vi "MLST.vi"(8 "error in (no error)":errorcluster, 10 "RemoteDirectory":string, 11 "FTP in":refnum<class "FTP.lvclass">) -> (0 "error out":errorcluster, 3 "FTP out":refnum<class "FTP.lvclass">)   [LabVIEW 2017, in "FTP_UpgradeCSMF.lvlib" / "FTP.lvclass"]
uses:
  FTP.lvclass
panel:
  out "Array":string[](array[string])
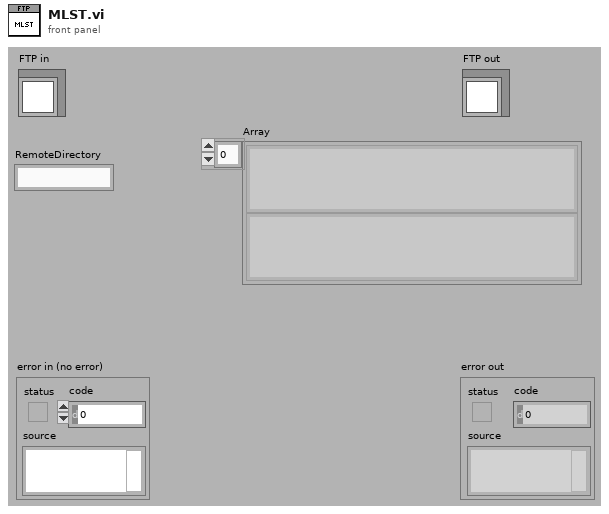
[diagram p1: front panel]
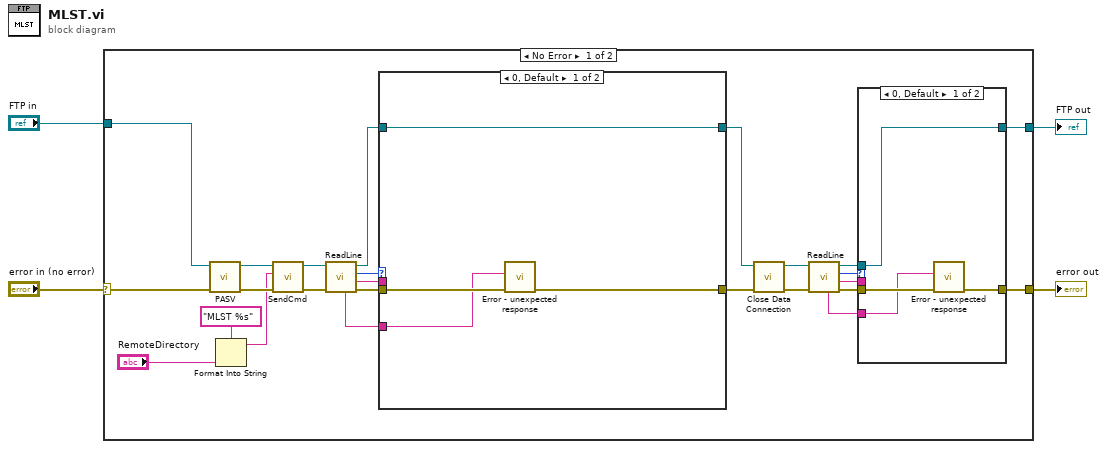
[diagram p0: block diagram]
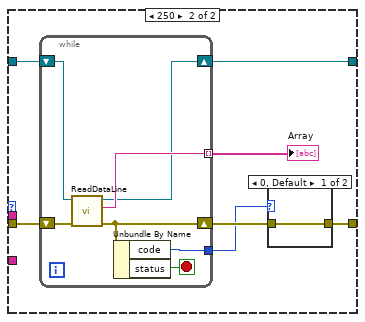
[diagram p3: hidden frame]
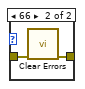
[diagram p4: hidden frame]
diagram:
  n1 = case shown="No Error" "error in (no error)" {
    selector: "error in (no error)" -> [w27 w58]
    tunnel: [w14 w58] -> w3
    tunnel: [w11 w57] -> w1
    tunnel: "FTP in" -> [w26 w57]
    frame No Error {
      n2 = call "PASV.vi"("error in (no error)"=w27, "FTP in"=w26) -> ("error out"=w24:errorcluster, "FTP out"=w25:refnum<class "FTP.lvclass">)  [unwired: 8 in]
      n3 = Format Into String(format string="MLST %s" ("cmd"), "RemoteDirectory") -> (resulting string=w8:string)  [unwired: 2 in, 1 out]
      n4 = call "SendCmd.vi"("error in (no error)"=w24, "cmd"=w8, "FTP in"=w25) -> ("error out"=w28:errorcluster, "FTP out"=w29:refnum<class "FTP.lvclass">)  [unwired: 7 in]
      n5 = call "ReadLine.vi"("error in (no error)"=w28, "FTP in"=w29) -> ("error out"=w23:errorcluster, "Line"=w21:string, "code"=w22:i32, "FTP out"=w20:refnum<class "FTP.lvclass">, "Full Line"=w5:string)  [unwired: 5 in]
      n6 = case shown="0, Default" w22 {
        tunnel: w23 -> [w38 w46]
        tunnel: w20 -> [w39 w45]
        tunnel: [w37 w43] -> w19
        tunnel: [w39 w42] -> w18
        tunnel: w21 -> [_ _]
        tunnel: w5 -> [w36 _]
        frame 0, Default {
          n7 = call "Error - unexpected response.vi"("error in (no error)"=w38, "Full Response"=w36) -> ("error out"=w37:errorcluster)  [unwired: 9 in]
        }
        frame 250 {
          n8 = while {
            tunnel: [w54] -> w44 mode=indexing
            shift-right: [w50] -> w41
            shift-left: w46 -> [w56]
            shift-right: [w51] -> w42
            shift-left: w45 -> [w55]
            tunnel: [w52] -> w40
            stop <- w53 stop-if-true
            n9 = call "ReadDataLine.vi"("error in (no error)"=w56, "FTP in"=w55) -> ("error out"=w50:errorcluster, "Data"=w54:string, "FTP out"=w51:refnum<class "FTP.lvclass">)  [unwired: 7 in]
            n10 = Unbundle By Name(w50) -> ("code"=w52:i32, "status"=w53:bool)
          }
          "Array" <- w44
          n11 = case shown="0, Default" w40 {
            tunnel: [w47 w49] -> w43
            tunnel: w41 -> [w47 w48]
            frame 0, Default {
            }
            frame 66 {
              n12 = call <vilib>:"Clear Errors.vi"("error in (no error)"=w48) -> ("error out"=w49:errorcluster)  [unwired: 5 in, 1 out]
            }
          }
        }
      }
      n13 = call "Close Data Connection.vi"("error in (no error)"=w19, "FTP in"=w18) -> ("error out"=w17:errorcluster, "FTP out"=w16:refnum<class "FTP.lvclass">)  [unwired: 8 in]
      n14 = call "ReadLine.vi"("error in (no error)"=w17, "FTP in"=w16) -> ("error out"=w15:errorcluster, "Line"=w10:string, "code"=w13:i32, "FTP out"=w12:refnum<class "FTP.lvclass">, "Full Line"=w6:string)  [unwired: 5 in]
      n15 = case shown="0, Default" w13 {
        tunnel: w15 -> [w32 w34]
        tunnel: [w31 w34] -> w14
        tunnel: w12 -> [w33 w35]
        tunnel: [w33 w35] -> w11
        tunnel: w10 -> [_ _]
        tunnel: w6 -> [w30 _]
        frame 0, Default {
          n16 = call "Error - unexpected response.vi"("error in (no error)"=w32, "Full Response"=w30) -> ("error out"=w31:errorcluster)  [unwired: 9 in]
        }
        frame 226 {
        }
      }
    }
    frame Error {
    }
  }
  "error out" <- w3
  "FTP out" <- w1
